vi "Get_Build_Data.vi"(8 "error in (no error)":errorcluster, 11 "Class in":refnum<class "AB_Build.lvclass">) -> (0 "error out":errorcluster, 2 "data":T1, 3 "Class out":refnum<class "AB_Build.lvclass">)   [LabVIEW 2020, in "AB_Build.lvclass"]
uses:
  <vilib>/AppBuilder/AB_Classes/Build/AB_Build.lvclass
  <vilib>/AppBuilder/AB_Classes/Build/AB_Build.ctl
  <vilib>/AppBuilder/AB_Classes/PreviewCache/PreviewCache.lvclass
  <vilib>/AppBuilder/AB_Classes/Destination/AB_Destination.lvclass
  <vilib>/AppBuilder/AB_Exclusion_Option.ctl
  <resource>/Framework/Providers/API/ItemRef.ctl
  <resource>/Framework/Providers/Common/provcom_ProgressBar_Events.ctl
  <resource>/Framework/Providers/API/mxLvBuildError.ctl
  <vilib>/AppBuilder/AB_Classes/Build/AB_Build.lvclass/AB_Build.ctl
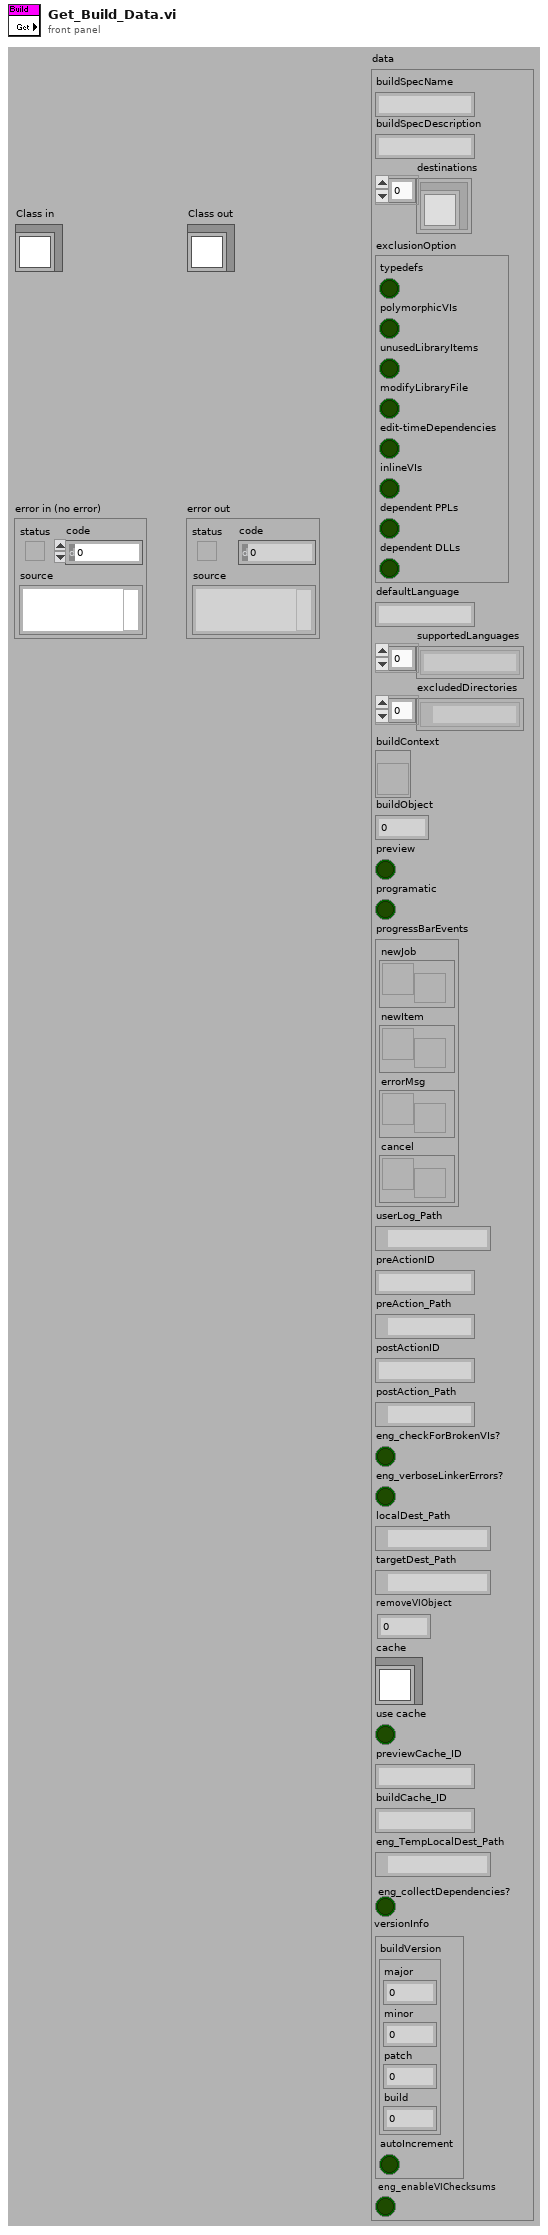
[diagram p1: front panel]
types:
  T1 = typedef "AB_Build.ctl" = cluster{"buildSpecName":string, "buildSpecDescription":string, "destinations":refnum<class "AB_Destination.lvclass">[], "exclusionOption":T2, "defaultLanguage":string, "supportedLanguages":string[], "excludedDirectories":path[], "buildContext":refnum<vi>, "buildObject":T3, "preview":bool, "programatic":bool, "progressBarEvents":T4, "userLog_Path":path, "preActionID":string, "preAction_Path":path, "postActionID":string, "postAction_Path":path, "eng_checkForBrokenVIs?":bool, "eng_verboseLinkerErrors?":bool, "localDest_Path":path, "targetDest_Path":path, "removeVIObject":u16, "cache":refnum<class "PreviewCache.lvclass">, "use cache":bool, "previewCache_ID":string, "buildCache_ID":string, "eng_TempLocalDest_Path":path, "eng_collectDependencies?":bool, "versionInfo":cluster{"buildVersion":cluster{"major":u16, "minor":u16, "patch":u16, "build":u16}, "autoIncrement":bool}, "eng_enableVIChecksums":bool}
  T2 = typedef "AB_Exclusion_Option.ctl" = cluster{"typedefs":bool, "polymorphicVIs":bool, "unusedLibraryItems":bool, "modifyLibraryFile":bool, "edit-timeDependencies":bool, "inlineVIs":bool, "dependent PPLs":bool, "dependent DLLs":bool}
  T3 = typedef "ItemRef.ctl" = u64
  T4 = typedef "provcom_ProgressBar_Events.ctl" = cluster{"newJob":refnum<user-event>, "newItem":refnum<user-event>, "errorMsg":T5, "cancel":refnum<user-event>}
  T5 = typedef "mxLvBuildError.ctl" = refnum<user-event>
  T6 = cluster{"buildVersion":cluster{"major":u16, "minor":u16, "patch":u16, "build":u16}, "autoIncrement":bool}
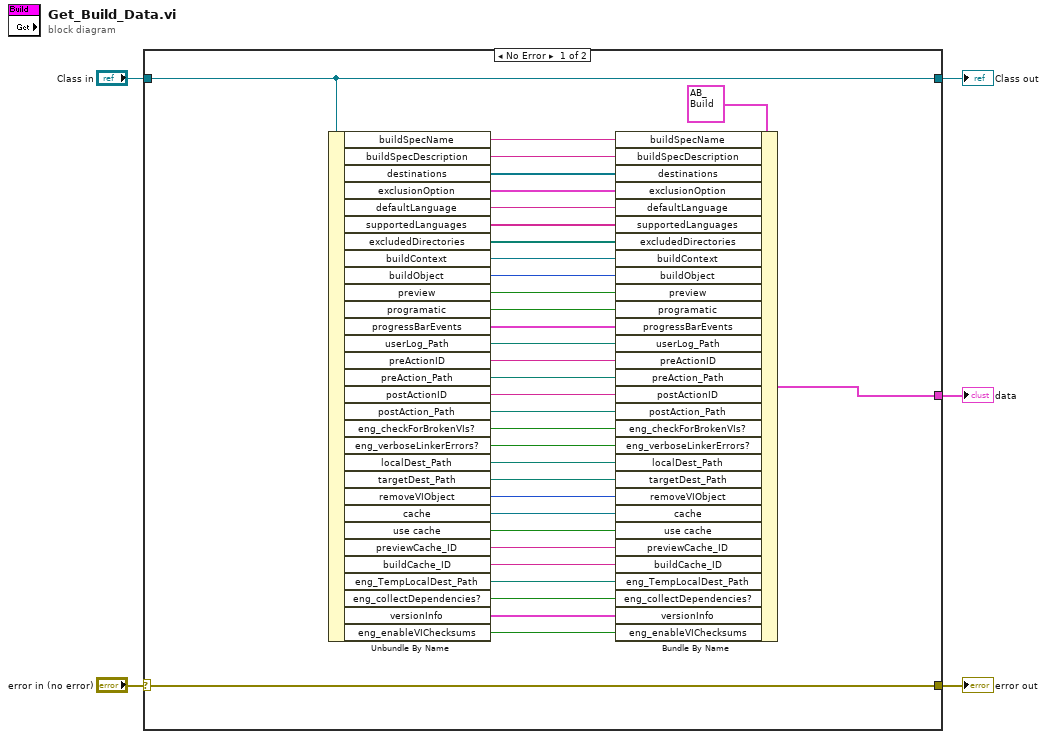
[diagram p0: block diagram]
diagram:
  n1 = case "Case" shown="No Error" "error in (no error)" {
    selector: "error in (no error)" -> [w39 w41]
    tunnel: [w39 w41] -> w4
    tunnel: [w30 w40] -> w2
    tunnel: "Class in" -> [w30 w40]
    tunnel: [w29 _] -> w1
    frame No Error {
      n2 = Unbundle By Name(w30) -> ("buildSpecName"=w28:string, "buildSpecDescription"=w25:string, "destinations"=w38:refnum<class "AB_Destination.lvclass">[], "exclusionOption"=w37:T2, "defaultLanguage"=w36:string, "supportedLanguages"=w35:string[], "excludedDirectories"=w34:path[], "buildContext"=w33:refnum<vi>, "buildObject"=w32:T3, "preview"=w31:bool, "programatic"=w27:bool, "progressBarEvents"=w26:T4, "userLog_Path"=w24:path, "preActionID"=w23:string, "preAction_Path"=w22:path, "postActionID"=w21:string, "postAction_Path"=w20:path, "eng_checkForBrokenVIs?"=w19:bool, "eng_verboseLinkerErrors?"=w18:bool, "localDest_Path"=w17:path, "targetDest_Path"=w16:path, "removeVIObject"=w15:u16, "cache"=w13:refnum<class "PreviewCache.lvclass">, "use cache"=w12:bool, "previewCache_ID"=w11:string, "buildCache_ID"=w9:string, "eng_TempLocalDest_Path"=w10:path, "eng_collectDependencies?"=w8:bool, "versionInfo"=w7:T6, "eng_enableVIChecksums"=w6:bool)
      n3 = Bundle By Name(cluster=T1 {"buildSpecName"="", "buildSpecDescription"="", "destinations"=[], "exclusionOption"={"typedefs"=FALSE, "polymorphicVIs"=FALSE, "unusedLibraryItems"=FALSE, "modifyLibraryFile"=FALSE, "edit-timeDependencies"=FALSE, "inlineVIs"=FALSE, "dependent PPLs"=FALSE, "dependent DLLs"=FALSE}, "defaultLanguage"="", "supportedLanguages"=[], "excludedDirectories"=[], "buildContext"=refnum, "buildObject"=0, "preview"=FALSE, "programatic"=FALSE, "progressBarEvents"={"newJob"=refnum, "newItem"=refnum, "errorMsg"=refnum, "cancel"=refnum}, "userLog_Path"=path "", "preActionID"="", "preAction_Path"=path "", "postActionID"="", "postAction_Path"=path "", "eng_checkForBrokenVIs?"=FALSE, "eng_verboseLinkerErrors?"=FALSE, "localDest_Path"=path "", "targetDest_Path"=path "", "removeVIObject"=0, "cache"=refnum, "use cache"=FALSE, "previewCache_ID"="", "buildCache_ID"="", "eng_TempLocalDest_Path"=path "", "eng_collectDependencies?"=FALSE, "versionInfo"={"buildVersion"={"major"=0, "minor"=0, "patch"=0, "build"=0}, "autoIncrement"=FALSE}, "eng_enableVIChecksums"=FALSE} ("buildSpecName"), "buildSpecName"=w28, "buildSpecDescription"=w25, "destinations"=w38, "exclusionOption"=w37, "defaultLanguage"=w36, "supportedLanguages"=w35, "excludedDirectories"=w34, "buildContext"=w33, "buildObject"=w32, "preview"=w31, "programatic"=w27, "progressBarEvents"=w26, "userLog_Path"=w24, "preActionID"=w23, "preAction_Path"=w22, "postActionID"=w21, "postAction_Path"=w20, "eng_checkForBrokenVIs?"=w19, "eng_verboseLinkerErrors?"=w18, "localDest_Path"=w17, "targetDest_Path"=w16, "removeVIObject"=w15, "cache"=w13, "use cache"=w12, "previewCache_ID"=w11, "buildCache_ID"=w9, "eng_TempLocalDest_Path"=w10, "eng_collectDependencies?"=w8, "versionInfo"=w7, "eng_enableVIChecksums"=w6) -> (w29:T1)
    }
    frame Error {
    }
  }
  "error out" <- w4
  "Class out" <- w2
  "data" <- w1
